vi "Bai3_6_C2.vi"() -> ()   [LabVIEW 2023]
panel:
  in  "Lines to Write 2":u16(ring) caption="Lines to Write" items=["0 - 7", "8 - 15", "16 - 23"]
  in  "Device Name 2":tag="Dev8" caption="Device Name den 2"
  in  "Device Name 1":tag="Dev8" caption="Device Name"
  in  "Lines to Write 1":u16(ring) caption="Lines to Write" items=["0 - 7", "8 - 15", "16 - 23"]
  in  "stop":bool
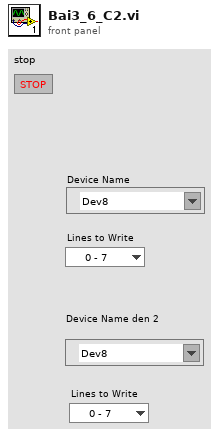
[diagram p1: front panel]
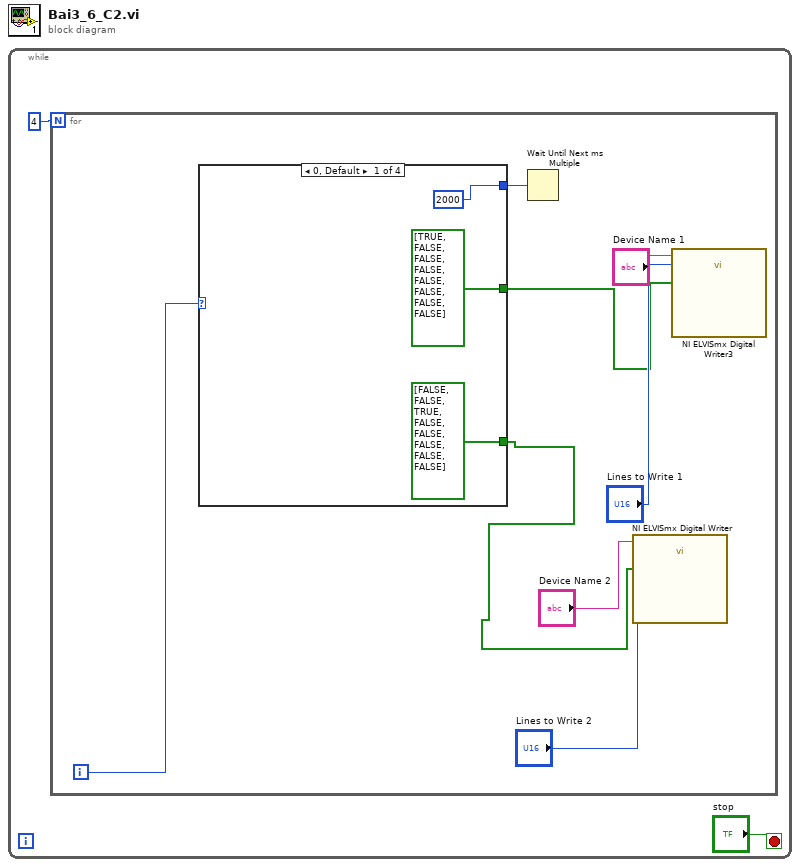
[diagram p0: block diagram]
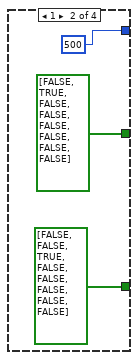
[diagram p2: hidden frame]
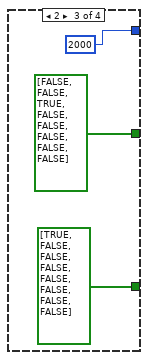
[diagram p3: hidden frame]
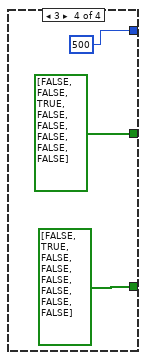
[diagram p4: hidden frame]
diagram:
  n1 = while {
    stop <- "stop" stop-if-true
    n2 = for {
      N: 4 -> [_]
      i -> [w6]
      n3 = case shown="0, Default" w6 {
        tunnel: [bool[] [TRUE, FALSE, FALSE, FALSE, FALSE, FALSE, FALSE, FALSE] bool[] [FALSE, TRUE, FALSE, FALSE, FALSE, FALSE, FALSE, FALSE] bool[] [FALSE, FALSE, TRUE, FALSE, FALSE, FALSE, FALSE, FALSE] bool[] [FALSE, FALSE, TRUE, FALSE, FALSE, FALSE, FALSE, FALSE]] -> w5
        tunnel: [bool[] [FALSE, FALSE, TRUE, FALSE, FALSE, FALSE, FALSE, FALSE] bool[] [FALSE, FALSE, TRUE, FALSE, FALSE, FALSE, FALSE, FALSE] bool[] [TRUE, FALSE, FALSE, FALSE, FALSE, FALSE, FALSE, FALSE] bool[] [FALSE, TRUE, FALSE, FALSE, FALSE, FALSE, FALSE, FALSE]] -> w4
        tunnel: [u32 2000 ("millisecond timer value") u32 500 ("millisecond timer value") u32 2000 ("millisecond timer value") u32 500 ("millisecond timer value")] -> w3
        frame 0, Default {
        }
        frame 1 {
        }
        frame 2 {
        }
        frame 3 {
        }
      }
      n4 = Wait Until Next ms Multiple(millisecond multiple=w3) -> ()  [unwired: 1 out]
      n5 = call "NI ELVISmx Digital Writer"("Device Name"="Device Name 2", "Lines to Write"="Lines to Write 2", "DO Lines"=w4) -> ()  [unwired: 16 in, 1 out]
      n6 = call "NI ELVISmx Digital Writer3"("Device Name"="Device Name 1", "Lines to Write"="Lines to Write 1", "DO Lines"=w5) -> ()  [unwired: 16 in, 1 out]
    }
  }
